vi "NumberArray_D.vi"(8 "error in (no error)":errorcluster, 10 "Start Number":i32, 11 "Array In":dbl[][](array[numeric])) -> (0 "error out":errorcluster, 3 "Array Out":dbl[][](array[numeric]))   [LabVIEW 2013]
doc: "This VI will number the 2D array with integers starting from \"Start Number\" (default = 1)"
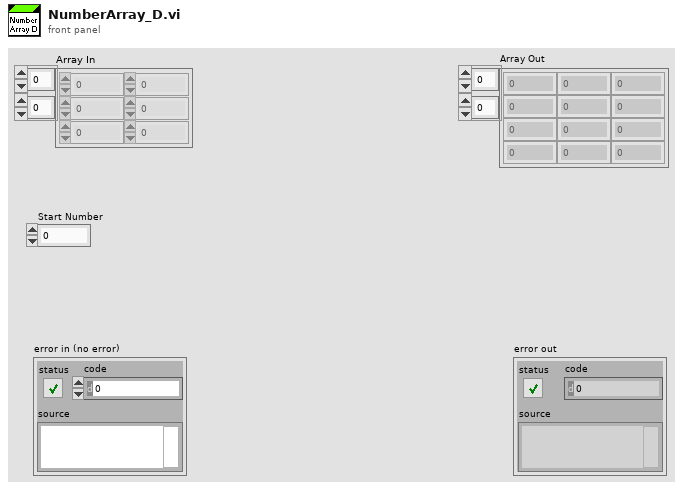
[diagram p1: front panel]
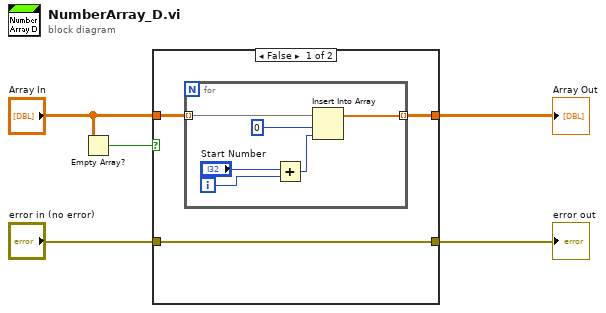
[diagram p0: block diagram]
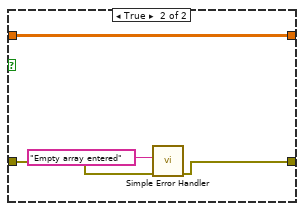
[diagram p2: hidden frame]
diagram:
  n1 = Empty Array?(array="Array In") -> (empty?=w3:bool)
  n2 = case shown="False" w3 {
    tunnel: "error in (no error)" -> [w8 w18]
    tunnel: [w8 w17] -> w4
    tunnel: "Array In" -> [w7 w15]
    tunnel: [w6 w15] -> w1
    frame False {
      n3 = for {
        tunnel: w7 -> [w14] mode=indexing
        tunnel: [w12] -> w6 mode=indexing
        i -> [w9]
        n4 = Add(x="Start Number", y=w9) -> (x+y=w11:i32)
        n5 = Insert Into Array(array=w14, index=0, new element=w11) -> (w12:dbl[])
      }
    }
    frame True {
      n6 = call <vilib>:"Simple Error Handler.vi"("error source (\" \")"="Empty array entered" ("error source (\" \")"), "error in (no error)"=w18) -> ("error out"=w17:errorcluster)  [unwired: 3 in, 4 out]
    }
  }
  "Array Out" <- w1
  "error out" <- w4
